vi "Shape.vi"(8 "error in (no error)":errorcluster, 10 "pShape.lvclass":refnum<class "pShape.lvclass">, 11 "pShape in":refnum<class "pShape.lvclass">) -> (0 "error out":errorcluster, 3 "pShape out":refnum<class "pShape.lvclass">)   [LabVIEW 2018, in "pShape.lvclass"]
uses:
  pShape.lvclass
  pShape.lvclass/pShape.ctl
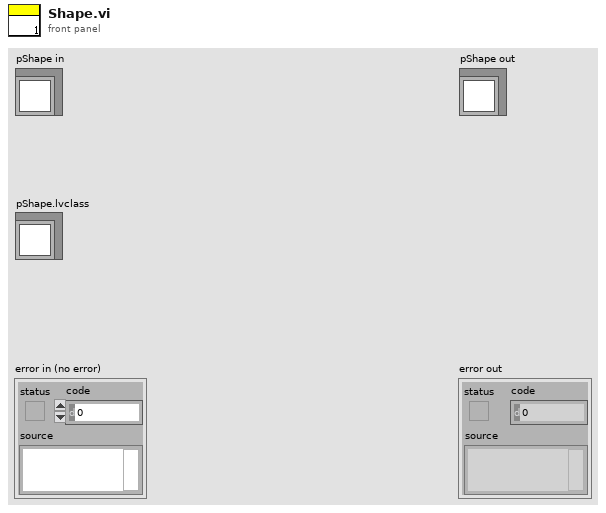
[diagram p1: front panel]
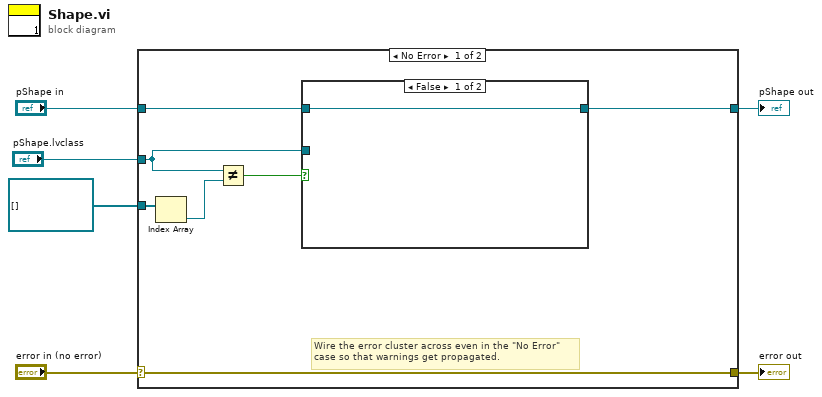
[diagram p0: block diagram]
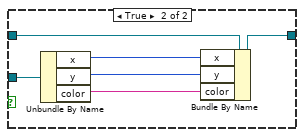
[diagram p2: hidden frame]
diagram:
  n1 = case shown="No Error" "error in (no error)" {
    selector: "error in (no error)" -> [w12 w22]
    tunnel: [w12 w22] -> w5
    tunnel: [w9 w21] -> w3
    tunnel: "pShape in" -> [w13 w21]
    tunnel: "pShape.lvclass" -> [w8 _]
    tunnel: refnum<class "pShape.lvclass">[] [] -> [w11 _]
    frame No Error {
      # "Wire the error cluster across even in the \"No Error\"\ncase so that warnings get propagated."
      n2 = Index Array(array=w11) -> (element=w10:refnum<class "pShape.lvclass">)  [unwired: 1 in]
      n3 = Not Equal?(x=w8, y=w10) -> (x != y?=w7:bool)
      n4 = case shown="False" w7 {
        tunnel: w13 -> [w14 w20]
        tunnel: [w14 w19] -> w9
        tunnel: w8 -> [_ w18]
        frame False {
        }
        frame True {
          n5 = Unbundle By Name(w18) -> ("x"=w17:i32, "y"=w16:i32, "color"=w15:string)
          n6 = Bundle By Name(cluster=w20, "x"=w17, "y"=w16, "color"=w15) -> (w19:refnum<class "pShape.lvclass">)
        }
      }
    }
    frame Error {
    }
  }
  "error out" <- w5
  "pShape out" <- w3
